vi "Unflatten from JSON.vi"(8 "error in (no error)":errorcluster, 9 "JSON Data":string, 10 "Version":string, 11 "Test Scope in":refnum<class "Test Scope.lvclass">) -> (0 "error out":errorcluster, 3 "Test Scope out":refnum<class "Test Scope.lvclass">)   [LabVIEW 2015, in "Test Scope.lvclass"]
uses:
  Test Scope.lvclass
  Test Scope.lvclass/Test Scope.ctl
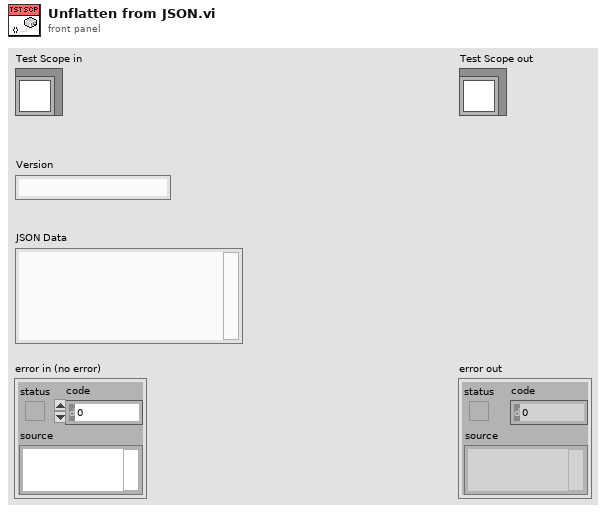
[diagram p1: front panel]
types:
  T1 = typedef "Test Scope.lvclass/JSON Data.ctl" = cluster{"V/div":dbl, "V Offset":dbl, "s/div":dbl, "s offset":dbl, "trigger level":dbl}
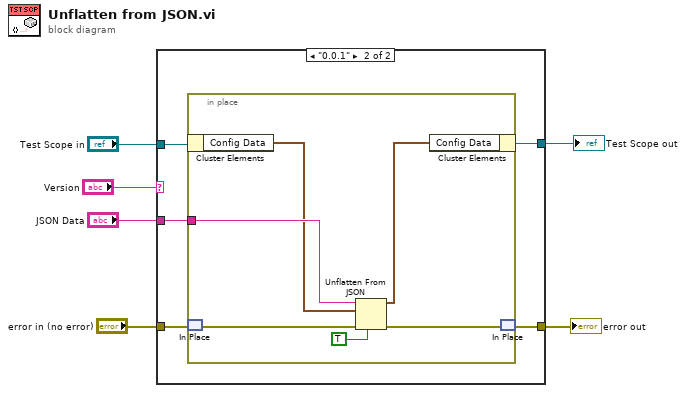
[diagram p0: block diagram]
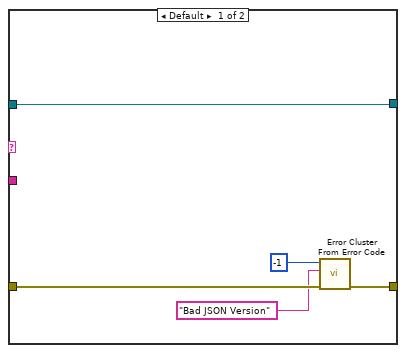
[diagram p2: hidden frame]
diagram:
  n1 = case shown="\"0.0.1\"" "Version" {
    tunnel: [w10 w13] -> w1
    tunnel: "error in (no error)" -> [w11 w15]
    tunnel: "JSON Data" -> [_ w14]
    tunnel: "Test Scope in" -> [w7 w16]
    tunnel: [w7 w12] -> w2
    frame Default {
      n2 = call <vilib>:"Error Cluster From Error Code.vi"("error in (no error)"=w11, "error message (\"\")"="Bad JSON Version" ("error message (\"\")"), "error code (0)"=-1) -> ("error out"=w10:errorcluster)  [unwired: 6 in]
    }
    frame "0.0.1" {
      n3 = in-place {
        in-place-border: w14 -> [w21]
        n4 = in-place-cluster #1(w16) -> ("Config Data"=w20:T1)
        n5 = in-place-match #2(w15) -> (w22:errorcluster)
        n6 = Unflatten From JSON(JSON string=w21, type and defaults=w20, default null elements? (F)=TRUE, error in (no error)=w22) -> (value=w19:T1, error out=w18:errorcluster)  [unwired: 3 in]
        n7 = in-place-cluster #1("Config Data"=w19) -> (w12:refnum<class "Test Scope.lvclass">)
        n8 = in-place-match #2(w18) -> (w13:errorcluster)
      }
    }
  }
  "error out" <- w1
  "Test Scope out" <- w2
